vi "Main.vi"() -> ()   [LabVIEW 2020]
doc: "Cet exemple de projet Mesure continue est basé sur le modèle Gestionnaire de messages dans une file d'attente.\n\nLa boucle de gestion d'événements génère des messages en fonction des actions sur l'interface utilisateur.\n\nLa boucle de gestion de messages traite les messages générés par la boucle de gestion d'événements ou par d'autres messages. Il y a aussi des sous-VIs de boucle de gestion de messages d'acquisition et d'enregistrement, ainsi qu'une boucle de mise à jour du graphe déroulant."
uses:
  Settings/Settings.ctl
  Acquisition/Hardware Configuration.ctl
  Acquisition/Signal Type.ctl
  Logging/Logging Configuration.ctl
  controls/UI Data.ctl
  controls/UI State.ctl
  support/Message Queue/Enqueue Message (Single).vi
  support/Message Queue/Enqueue Message (Array).vi
  <vilib>/Utility/error.llb/Error Cluster From Error Code.vi
  <vilib>/ErrorRing/Error Ring.xnode
  Acquisition/Acquisition.lvlib
  Logging/Logging.lvlib
  Settings/Settings.lvlib
  support/User Event - Stop/User Event - Stop.lvlib
  support/Message Queue/Message Queue.lvlib
  Settings/Settings Dialog.vi
panel:
  in  "Panneaux":T1(tab)
  in  "Param status":bool
  out "Données":waveform(dbl)[](graph)
  out "État":string
  in  "Quitter":bool
  in  "Arrêter":bool
  in  "Démarrer":bool
  in  "Paramètres":bool
  # "MAPA Tech"
  # "MAPA Tech"
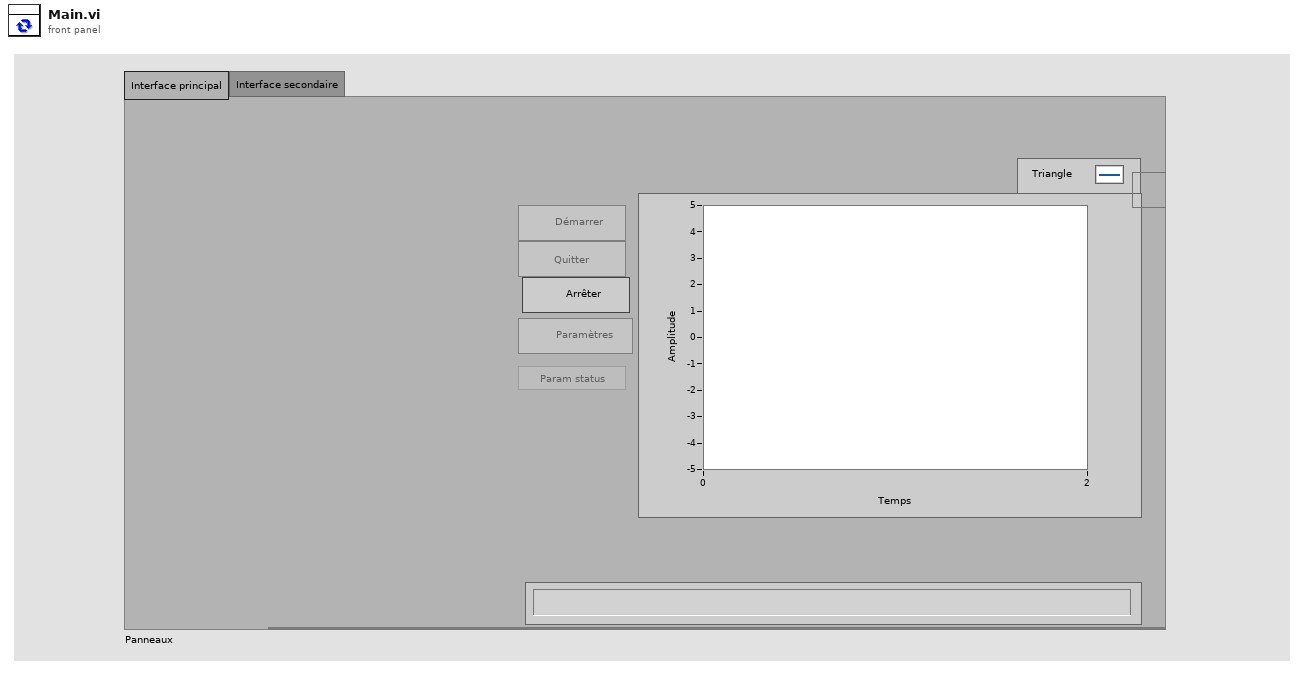
[diagram p1: front panel]
types:
  T1 = enum32{"Interface principal", "Interface secondaire"}
  T2 = typedef "UI State.ctl" = enum16{"Idle", "Acquiring and Logging", "Waiting for Exit", "Waiting for Exit (Acq Stopped)", "Waiting for Exit (Log Stopped)", "Waiting for Stop", "Waiting for Stop (Acq Stopped)", "Waiting for Stop (Log Stopped)"}
  T3 = typedef "UI Data.ctl" = cluster{"Réf. de Démarrer":refnum<vi>, "Réf. d'Arrêter":refnum<vi>, "Réf. de Paramètres":refnum<vi>, "Réf. de Quitter":refnum<vi>, "Réf. d'état":refnum<vi>, "Réf. de données":refnum<vi>, "Ref. Moyennage sélectionneur":refnum<vi>, "Ref. Param status":refnum<vi>}
  T4 = typedef "Settings.lvlib/Settings.ctl" = cluster{"Configuration du matériel":T5, "Configuration de l'enregistrement":T7, "Mode de longueur d'onde":cluster{"Choix du mode":bool, "Commande numérique":dbl}}
  T5 = typedef "Acquisition.lvlib/Hardware Configuration.ctl" = cluster{"Refnum de matériel <À remplacer>":string, "Type de signal <À remplacer>":T6}
  T6 = typedef "Acquisition.lvlib/Signal Type.ctl" = enum16{"Sine Wave", "Square with Noise", "Signal triangulaire", "Simulation DAQ"}
  T7 = typedef "Logging.lvlib/Logging Configuration.ctl" = cluster{"Chemin de base du fichier journal":path, "Référence de fichier TDMS":refnum<k34>}
  T8 = cluster{"état":bool, "code":i32, "source":string}
  T9 = typedef "Message Queue.lvlib/All Message Queues.ctl" = cluster{"IU":refnum<queue>, "Acquisition":refnum<queue>, "Enregistrement":refnum<queue>}
  T10 = cluster{"Choix du mode":bool, "Commande numérique":dbl}
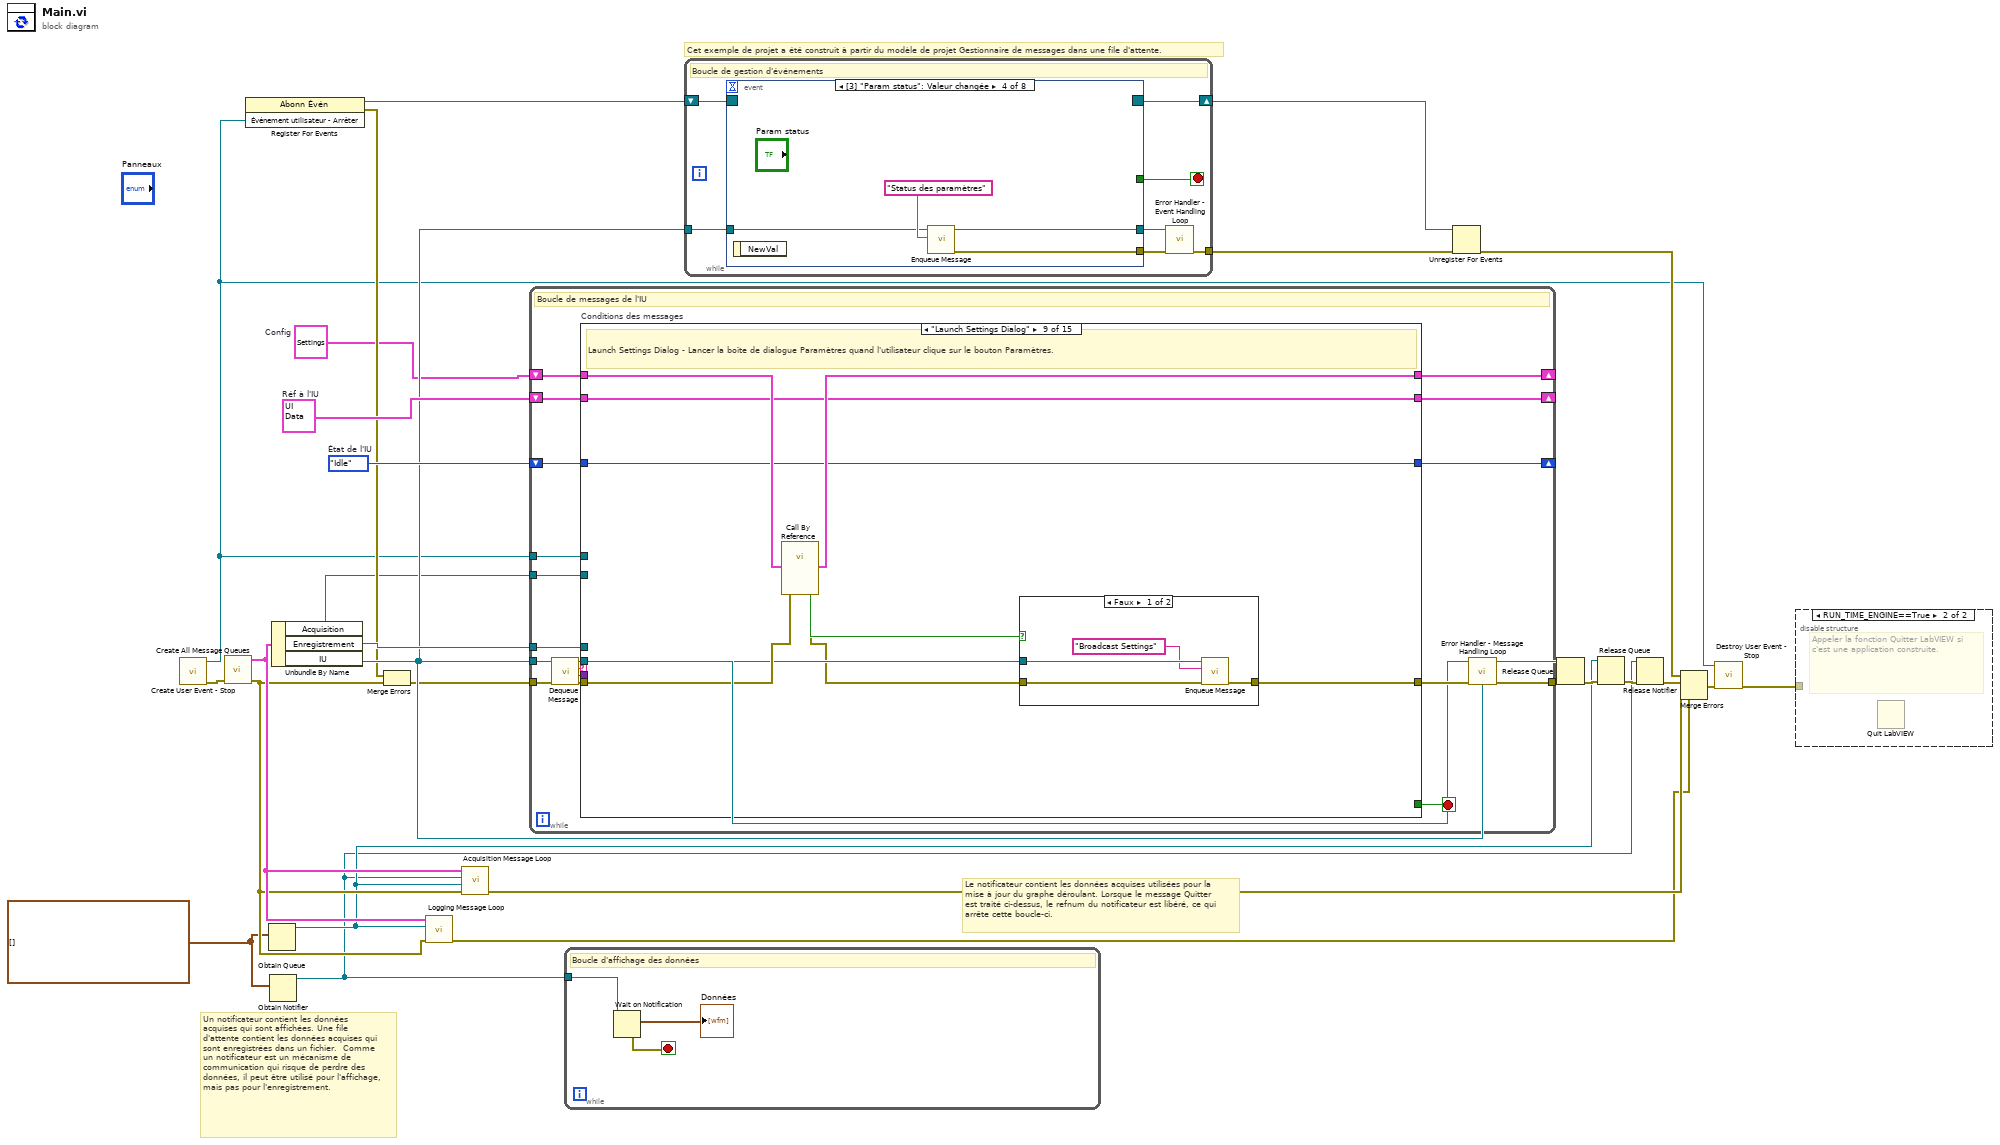
[diagram p0: block diagram]
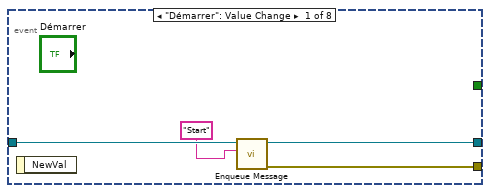
[diagram p3: hidden frame]
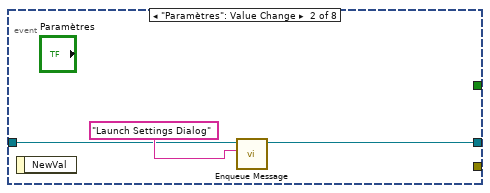
[diagram p4: hidden frame]
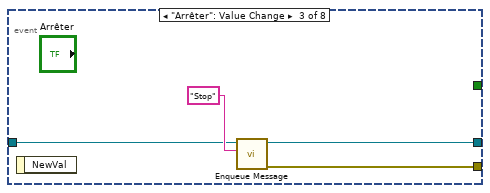
[diagram p5: hidden frame]
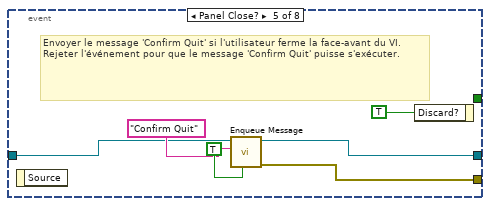
[diagram p6: hidden frame]
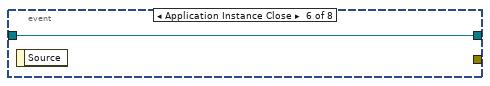
[diagram p7: hidden frame]
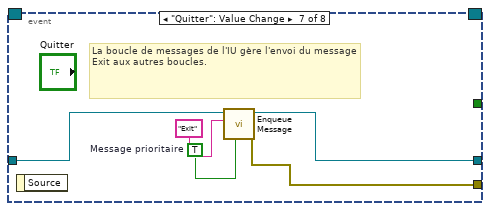
[diagram p8: hidden frame]
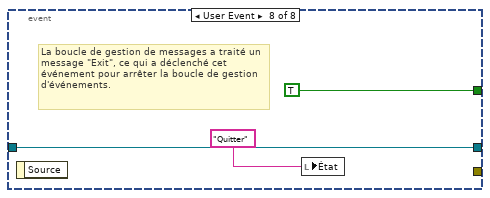
[diagram p9: hidden frame]
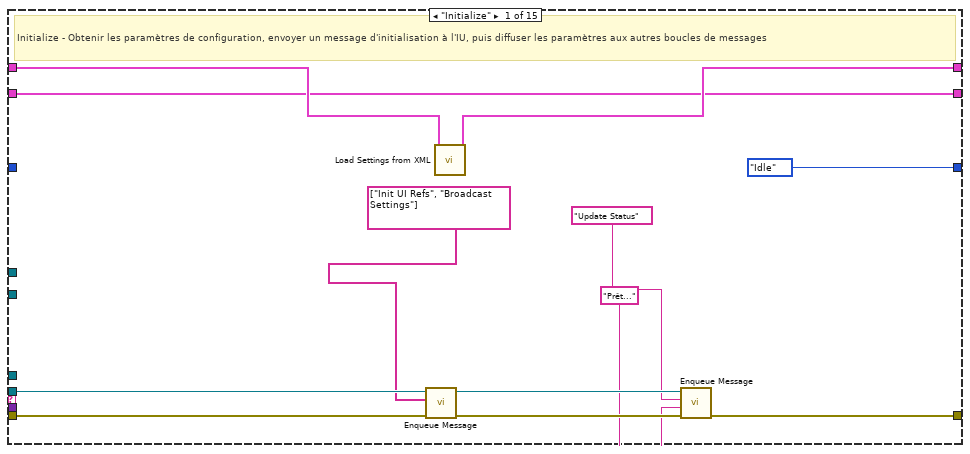
[diagram p10: hidden frame]
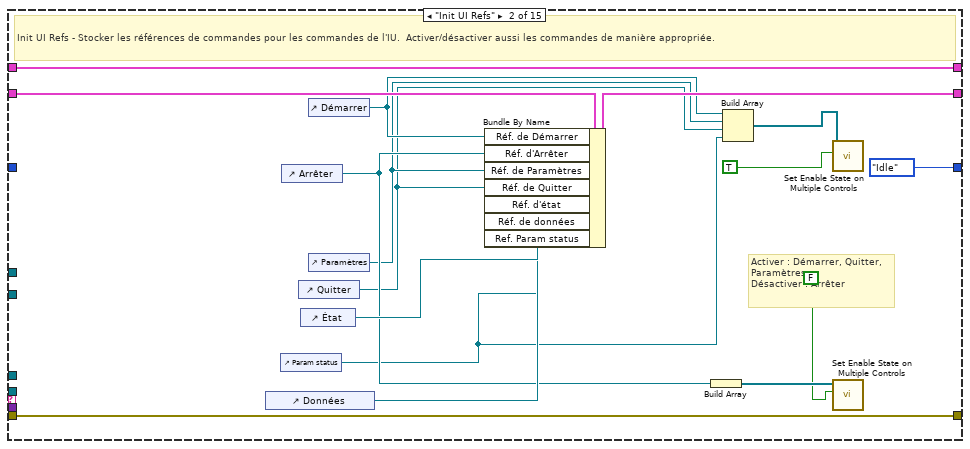
[diagram p11: hidden frame]
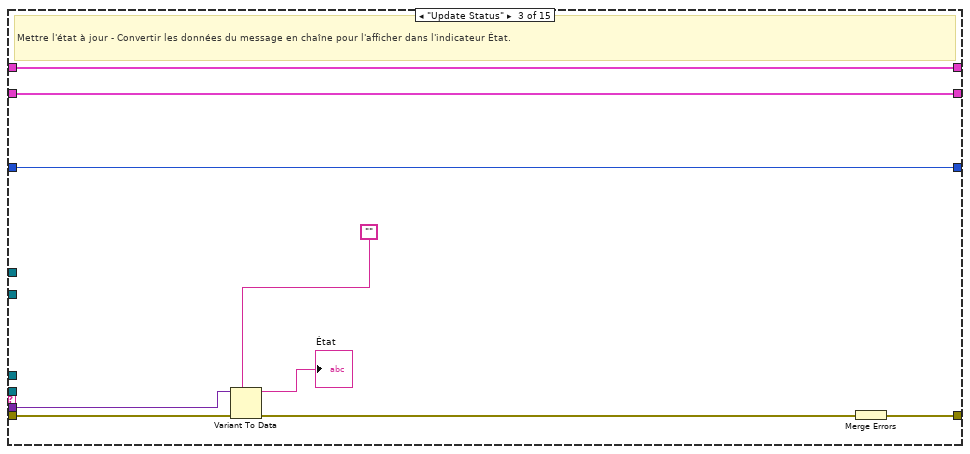
[diagram p12: hidden frame]
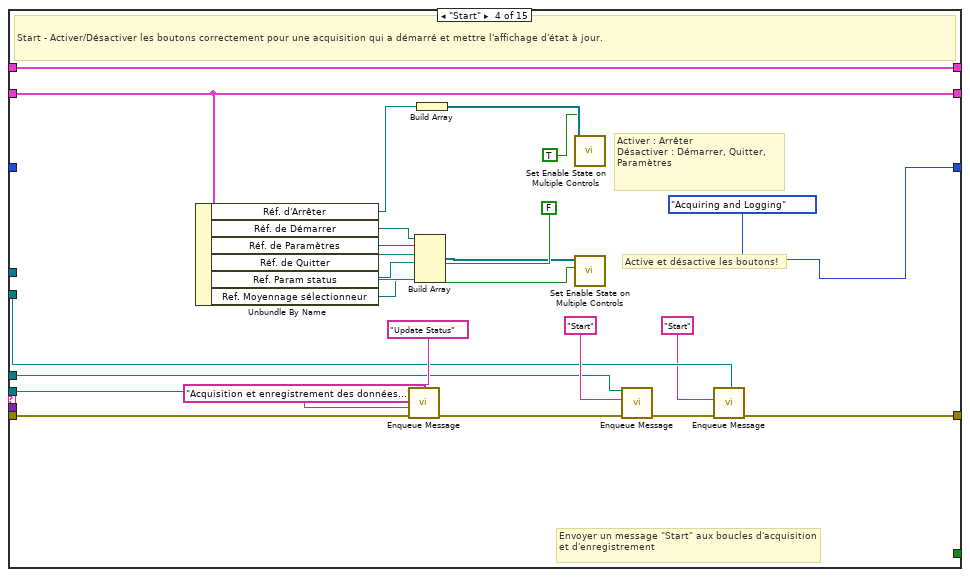
[diagram p13: hidden frame]
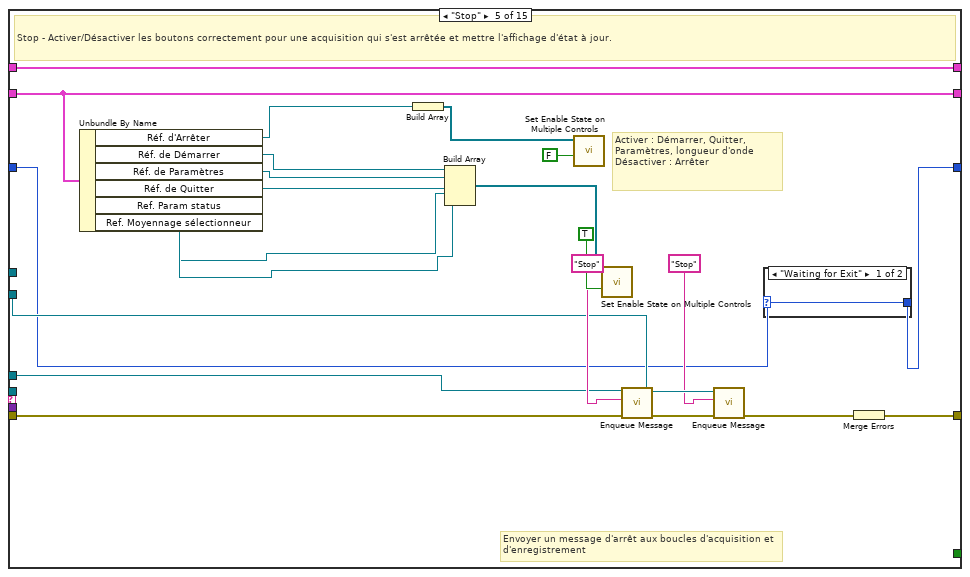
[diagram p14: hidden frame]
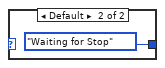
[diagram p15: hidden frame]
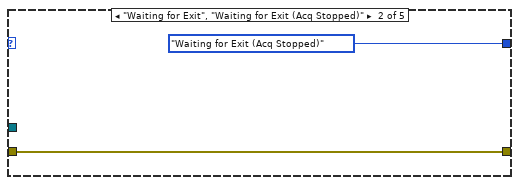
[diagram p17: hidden frame]
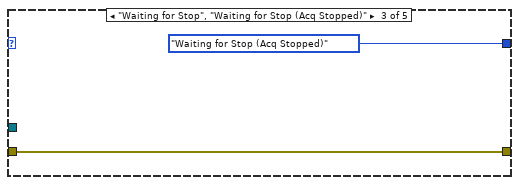
[diagram p18: hidden frame]
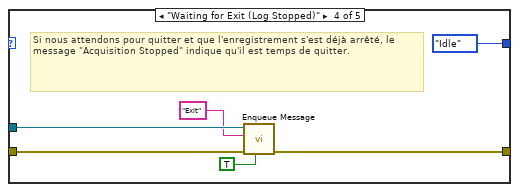
[diagram p19: hidden frame]
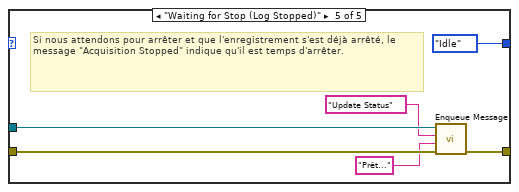
[diagram p20: hidden frame]
diagram:
  w16 = UI_State."Idle"  # État de l'IU
  w2 = waveform(dbl)[] []
  w18 = T3 {"Réf. de Démarrer"=refnum, "Réf. d'Arrêter"=refnum, "Réf. de Paramètres"=refnum, "Réf. de Quitter"=refnum, "Réf. d'état"=refnum, "Réf. de données"=refnum, "Ref. Moyennage sélectionneur"=refnum, "Ref. Param status"=refnum}  # Réf à l'IU
  w1 = T4 {"Configuration du matériel"={"Refnum de matériel <À remplacer>"="", "Type de signal <À remplacer>"=enum."Simulation DAQ"}, "Configuration de l'enregistrement"={"Chemin de base du fichier journal"=path "", "Référence de fichier TDMS"=refnum}, "Mode de longueur d'onde"={"Choix du mode"=TRUE, "Commande numérique"=15.0}}  # Config
  # "Cet exemple de projet a été construit à partir du modèle de projet Gestionnaire de messages dans une file d'attente."
  # "Un notificateur contient les données acquises qui sont affichées. Une file d'attente contient les données acquises qui sont enregistrées dans un fichier.  Comme un notificateur est un mécanisme de communication qui risque de perdre des données, il peut être utilisé pour l'affichage, mais pas pour l'enregistrement."
  # "Le notificateur contient les données acquises utilisées pour la mise à jour du graphe déroulant. Lorsque le message Quitter est traité ci-dessus, le refnum du notificateur est libéré, ce qui arrête cette boucle-ci."
  n1 = call "Create User Event - Stop.vi"() -> ("error out"=w24:T8, "Événement utilisateur - Arrêter"=w3:refnum<user-event>)  [unwired: 10 in]
  n2 = call "Create All Message Queues.vi"("error in (no error)"=w24) -> ("error out"=w21:T8, "Files d'attente de messages en sortie"=w23:T9)  [unwired: 9 in]
  n3 = register-events(w3) -> (reference out=w7:refnum<event-registration>, error out=w5:errorcluster)  [unwired: 2 in]
  n4 = Obtain Queue(element data type=w2) -> (queue out=w9:refnum<queue>)  [unwired: 4 in, 2 out]
  n5 = Obtain Notifier(notification data type=w2) -> (notifier out=w8:refnum<notifier>)  [unwired: 3 in, 2 out]
  n6 = Unbundle By Name(w23) -> ("Acquisition"=w4:refnum<queue>, "Enregistrement"=w17:refnum<queue>, "IU"=w14:refnum<queue>)
  n7 = Merge Errors(w5, w21) -> (w6:errorcluster)
  n8 = call "Logging Message Loop.vi"("error in (no error)"=w21, "File d'attente de données"=w9, "Files d'attente de messages"=w23) -> ("error out"=w22:T8)  [unwired: 8 in]
  n9 = call "Acquisition Message Loop.vi"("error in (no error)"=w21, "File d'attente de données"=w9, "Notificateur de données"=w8, "Files d'attente de messages"=w23) -> ("error out"=w25:T8)  [unwired: 7 in]
  n10 = while {
    tunnel: w14 -> [w39]
    tunnel: w3 -> [w44]
    shift-right: [w38] -> _
    shift-left: w1 -> [w37]
    shift-right: [w35] -> _
    shift-left: w18 -> [w36]
    tunnel: w4 -> [w34]
    tunnel: w17 -> [w33]
    shift-right: [w28] -> _
    shift-left: w16 -> [w29]
    tunnel: w6 -> [w43]
    tunnel: [w32] -> w27
    stop <- w45 stop-if-true
    # "Boucle de messages de l'IU"
    n11 = call "Dequeue Message.vi"("error in (no error)"=w43, "File d'attente de messages"=w39) -> ("error out"=w42:T8, "Données de message"=w40:variant, "Message"=w41:string, "File d'attente de message dup."=w30:refnum<queue>)  [unwired: 6 in]
    n12 = case "Conditions des messages" shown="\"Launch Settings Dialog\"" w41 {
      selector: w41 -> [_ _ _ _ _ _ _ _ _ _ _ _ _ _ w285]
      tunnel: w30 -> [w49 _ _ w106 _ w133 w158 _ w200 _ w221 _ _ w272 _]
      tunnel: w42 -> [w48 w73 w81 w105 w127 w134 w159 w188 w202 w209 w220 w249 w266 w276 _]
      tunnel: [w53 w73 w82 w92 w128 w131 w156 w194 w195 w212 w219 w259 w265 w275 w284] -> w31
      tunnel: [_ _ _ _ _ _ _ _ _ _ _ TRUE _ _ _] -> w45
      tunnel: w40 -> [_ _ w80 _ _ _ _ _ _ w213 _ w247 _ _ _]
      tunnel: w44 -> [_ _ _ _ _ _ _ _ _ _ _ w260 _ _ _]
      tunnel: [w56 w72 w76 w104 w126 w137 w162 w192 w199 w217 w224 w258 w264 w270 w288] -> w38
      tunnel: w37 -> [w57 w72 w76 w104 w126 w137 w162 w192 w203 w217 w224 w258 w264 w270 w288]
      tunnel: w36 -> [w50 w71 w75 w101 w125 w136 w161 w187 w197 w216 w223 w257 w263 w274 w287]
      tunnel: [w50 w68 w75 w101 w125 w136 w161 w187 w197 w216 w223 w257 w263 w274 w287] -> w35
      tunnel: w34 -> [_ _ _ w91 w118 _ _ w186 _ _ _ w256 _ _ _]
      tunnel: w33 -> [_ _ _ w94 w121 _ _ w181 _ _ _ w255 _ _ _]
      tunnel: w29 -> [_ _ w74 _ w115 w135 w160 w185 w196 w211 w222 _ w262 _ w286]
      tunnel: [UI_State."Idle" ("UI State") UI_State."Idle" ("UI State") w74 UI_State."Acquiring and Logging" ("UI State") w116 w132 w157 w185 w196 w211 w218 UI_State."Idle" ("UI State") w262 UI_State."Acquiring and Logging" ("UI State") w286] -> w28
      frame "Initialize" {
        # "Initialize - Obtenir les paramètres de configuration, envoyer un message d'initialisation à l'IU, puis diffuser les paramètres aux autres boucles de messages"
        n13 = call-poly "Enqueue Message.vi"("error in (no error)"=w48, "Tableau de messages"=string[] ["Init UI Refs", "Broadcast Settings"], "File d'attente de messages"=w49) -> ("error out"=w55:T8, "File d'attente de message dup."=w54:refnum<queue>)  [unwired: 7 in]
        n14 = call "Load Settings from XML.vi"("Paramètres en entrée"=w57) -> ("Paramètres en sortie"=w56:T4)  [unwired: 9 in, 1 out]
        n15 = call-poly "Enqueue Message.vi"("error in (no error)"=w55, "Données de message"="Prêt..." ("Ready..."), "Message"="Update Status", "File d'attente de messages"=w54) -> ("error out"=w53:T8)  [unwired: 6 in, 1 out]
      }
      frame "Init UI Refs" {
        # "Activer : Démarrer, Quitter, Paramètres\nDésactiver : Arrêter"
        # "Init UI Refs - Stocker les références de commandes pour les commandes de l'IU.  Activer/désactiver aussi les commandes de manière appropriée."
        n16 = control-ref of="Données"() -> (w69:refnum<vi>)
        n17 = control-ref of="Param status"() -> (w58:refnum<vi>)
        n18 = control-ref of="Arrêter"() -> (w63:refnum<vi>)
        n19 = control-ref of="Quitter"() -> (w60:refnum<vi>)
        n20 = control-ref of="État"() -> (w70:refnum<vi>)
        n21 = control-ref of="Démarrer"() -> (w62:refnum<vi>)
        n22 = control-ref of="Paramètres"() -> (w61:refnum<vi>)
        n23 = Bundle By Name(cluster=w71, "Réf. de Démarrer"=w62, "Réf. d'Arrêter"=w63, "Réf. de Paramètres"=w61, "Réf. de Quitter"=w60, "Réf. d'état"=w70, "Réf. de données"=w69, "Ref. Param status"=w58) -> (w68:T3)
        n24 = Build Array(w63) -> (w65:refnum<vi>[])
        n25 = Build Array(w62, w61, w60, w58) -> (w66:refnum<vi>[])
        n26 = call "Set Enable State on Multiple Controls.vi"("Activé ?"=TRUE ("Enable?"), "Commandes"=w66) -> ()  [unwired: 10 in]
        n27 = call "Set Enable State on Multiple Controls.vi"("Activé ?"=FALSE ("Enable?"), "Commandes"=w65) -> ()  [unwired: 10 in]
      }
      frame "Update Status" {
        # "Mettre l'état à jour - Convertir les données du message en chaîne pour l'afficher dans l'indicateur État."
        n28 = Variant To Data(error in=w81, type="" ("Empty String Constant"), Variant=w80) -> (data=→"État":string, error out=w78:errorcluster)
        n29 = Merge Errors(w78) -> (w82:errorcluster)
      }
      frame "Start" {
        # "Active et désactive les boutons!"
        # "Envoyer un message \"Start\" aux boucles d'acquisition et d'enregistrement"
        # "Activer : Arrêter\nDésactiver : Démarrer, Quitter, Paramètres"
        # "Start - Activer/Désactiver les boutons correctement pour une acquisition qui a démarré et mettre l'affichage d'état à jour."
        n30 = Unbundle By Name(w101) -> ("Réf. d'Arrêter"=w83:refnum<vi>, "Réf. de Démarrer"=w84:refnum<vi>, "Réf. de Paramètres"=w85:refnum<vi>, "Réf. de Quitter"=w88:refnum<vi>, "Ref. Param status"=w87:refnum<vi>, "Ref. Moyennage sélectionneur"=w86:refnum<vi>)
        n31 = call-poly "Enqueue Message.vi"("error in (no error)"=w105, "Données de message"="Acquisition et enregistrement des données..." ("Acquiring and Logging..."), "Message"="Update Status", "File d'attente de messages"=w106) -> ("error out"=w96:T8)  [unwired: 6 in, 1 out]
        n32 = Build Array(w84, w85, w85, w88, w87, w86) -> (w99:refnum<vi>[])
        n33 = Build Array(w83) -> (w98:refnum<vi>[])
        n34 = call "Set Enable State on Multiple Controls.vi"("Activé ?"=TRUE ("Enable?"), "Commandes"=w98) -> ()  [unwired: 10 in]
        n35 = call "Set Enable State on Multiple Controls.vi"("Activé ?"=FALSE ("Enable?"), "Commandes"=w99) -> ()  [unwired: 10 in]
        n36 = call-poly "Enqueue Message.vi"("error in (no error)"=w96, "Message"="Start", "File d'attente de messages"=w94) -> ("error out"=w93:T8)  [unwired: 7 in, 1 out]
        n37 = call-poly "Enqueue Message.vi"("error in (no error)"=w93, "Message"="Start", "File d'attente de messages"=w91) -> ("error out"=w92:T8)  [unwired: 7 in, 1 out]
      }
      frame "Stop" {
        # "Envoyer un message d'arrêt aux boucles d'acquisition et d'enregistrement"
        # "Activer : Démarrer, Quitter, Paramètres, longueur d'onde\nDésactiver : Arrêter"
        # "Stop - Activer/Désactiver les boutons correctement pour une acquisition qui s'est arrêtée et mettre l'affichage d'état à jour."
        n38 = Unbundle By Name(w125) -> ("Réf. d'Arrêter"=w107:refnum<vi>, "Réf. de Démarrer"=w108:refnum<vi>, "Réf. de Paramètres"=w109:refnum<vi>, "Réf. de Quitter"=w110:refnum<vi>, "Ref. Param status"=w111:refnum<vi>, "Ref. Moyennage sélectionneur"=w112:refnum<vi>)
        n39 = Build Array(w107) -> (w113:refnum<vi>[])
        n40 = Build Array(w108, w109, w110, w111, w112) -> (w114:refnum<vi>[])
        n41 = call "Set Enable State on Multiple Controls.vi"("Activé ?"=FALSE ("Enable?"), "Commandes"=w113) -> ()  [unwired: 10 in]
        n42 = call "Set Enable State on Multiple Controls.vi"("Activé ?"=TRUE ("Enable?"), "Commandes"=w114) -> ()  [unwired: 10 in]
        n43 = call-poly "Enqueue Message.vi"("error in (no error)"=w127, "Message"="Stop", "File d'attente de messages"=w121) -> ("error out"=w120:T8)  [unwired: 7 in, 1 out]
        n44 = call-poly "Enqueue Message.vi"("error in (no error)"=w120, "Message"="Stop", "File d'attente de messages"=w118) -> ("error out"=w119:T8)  [unwired: 7 in, 1 out]
        n45 = case shown="\"Waiting for Exit\"" w115 {
          selector: w115 -> [w129 _]
          tunnel: [w129 UI_State."Waiting for Stop" ("UI State")] -> w116
          frame "Waiting for Exit" {
          }
          frame Default {
          }
        }
        n46 = Merge Errors(w119) -> (w128:errorcluster)
      }
      frame "Acquisition Stopped" {
        # "Logique déterminant quelle action entreprendre quand l'acquisition s'est arrêtée."
        n47 = case shown="Par défaut" w135 {
          selector: w135 -> [w139 _ _ _ _]
          tunnel: w134 -> [w138 w141 w143 w149 w155]
          tunnel: w133 -> [_ _ _ w147 w152]
          tunnel: [w139 UI_State."Waiting for Exit (Acq Stopped)" ("UI State") UI_State."Waiting for Stop (Acq Stopped)" ("UI State") UI_State."Idle" ("UI State") UI_State."Idle" ("UI State")] -> w132
          tunnel: [w138 w141 w143 w148 w153] -> w131
          frame Default {
          }
          frame "Waiting for Exit", "Waiting for Exit (Acq Stopped)" {
          }
          frame "Waiting for Stop", "Waiting for Stop (Acq Stopped)" {
          }
          frame "Waiting for Exit (Log Stopped)" {
            # "Si nous attendons pour quitter et que l'enregistrement s'est déjà arrêté, le message \"Acquisition Stopped\" indique qu'il est temps de quitter."
            n48 = call-poly "Enqueue Message.vi"("Message prioritaire ? (F)"=TRUE ("Priority Message? (F)"), "error in (no error)"=w149, "Message"="Exit", "File d'attente de messages"=w147) -> ("error out"=w148:T8)  [unwired: 6 in, 1 out]
          }
          frame "Waiting for Stop (Log Stopped)" {
            # "Si nous attendons pour arrêter et que l'enregistrement s'est déjà arrêté, le message \"Acquisition Stopped\" indique qu'il est temps d'arrêter."
            n49 = call-poly "Enqueue Message.vi"("error in (no error)"=w155, "Données de message"="Prêt..." ("Ready..."), "Message"="Update Status", "File d'attente de messages"=w152) -> ("error out"=w153:T8)  [unwired: 6 in, 1 out]
          }
        }
      }
      frame "Logging Stopped" {
        # "Logique déterminant quelle action entreprendre quand l'enregistrement s'est arrêté."
        n50 = case shown="\"Waiting for Stop (Acq Stopped)\"" w160 {
          selector: w160 -> [w164 _ _ _ _]
          tunnel: w159 -> [w163 w166 w168 w174 w177]
          tunnel: w158 -> [_ _ _ w172 w176]
          tunnel: [w164 UI_State."Waiting for Exit (Log Stopped)" ("UI State") UI_State."Waiting for Stop (Log Stopped)" ("UI State") UI_State."Idle" ("UI State") UI_State."Idle" ("UI State")] -> w157
          tunnel: [w163 w166 w168 w173 w175] -> w156
          frame Default {
          }
          frame "Waiting for Exit", "Waiting for Exit (Log Stopped)" {
          }
          frame "Waiting for Stop", "Waiting for Stop (Log Stopped)" {
          }
          frame "Waiting for Exit (Acq Stopped)" {
            # "Si nous attendons pour quitter et que l'acquisition s'est déjà arrêtée, le message \"Logging Stopped\" indique qu'il est temps de quitter."
            n51 = call-poly "Enqueue Message.vi"("Message prioritaire ? (F)"=TRUE ("Priority Message? (F)"), "error in (no error)"=w174, "Message"="Exit", "File d'attente de messages"=w172) -> ("error out"=w173:T8)  [unwired: 6 in, 1 out]
          }
          frame "Waiting for Stop (Acq Stopped)" {
            # "Si nous attendons pour arrêter et que l'acquisition s'est déjà arrêtée, le message \"Logging Stopped\" indique qu'il est temps d'arrêter."
            n52 = call-poly "Enqueue Message.vi"("error in (no error)"=w177, "Données de message"="Prêt..." ("Ready..."), "Message"="Update Status", "File d'attente de messages"=w176) -> ("error out"=w175:T8)  [unwired: 6 in, 1 out]
          }
        }
      }
      frame "Broadcast settings" {
        w182 = "Update Settings" ("Message")
        # "Broadcast settings - Envoyer le message 'Update Settings' aux boucles de messages d'enregistrement et d'acquisition."
        n53 = Unbundle By Name(w192) -> ("Configuration du matériel"=w191:T5, "Configuration de l'enregistrement"=w190:T7, "Mode de longueur d'onde"=w184:T10)
        n54 = call-poly "Enqueue Message.vi"("Données de message"=w191, "Message"=w182, "File d'attente de messages"=w186) -> ("error out"=w193:T8)  [unwired: 7 in, 1 out]
        n55 = call-poly "Enqueue Message.vi"("Données de message"=w184, "Message"=w182, "File d'attente de messages"=w181) -> ("error out"=w183:T8)  [unwired: 7 in, 1 out]
        n56 = call-poly "Enqueue Message.vi"("error in (no error)"=w193, "Données de message"=w190, "Message"=w182, "File d'attente de messages"=w181) -> ("error out"=w189:T8)  [unwired: 6 in, 1 out]
        n57 = Merge Errors(w183, w189, w188) -> (w194:errorcluster)
      }
      frame "Launch Settings Dialog" {
        # "Launch Settings Dialog - Lancer la boîte de dialogue Paramètres quand l'utilisateur clique sur le bouton Paramètres."
        n58 = call-by-ref "?"("error in (no error)"=w202, "Paramètres en entrée"=w203) -> ("error out"=w198:T8, "Annulation ?"=w201:bool, "Paramètres en sortie"=w199:T4)  [unwired: 8 in, 3 out]
        n59 = case shown="Faux" w201 {
          tunnel: w200 -> [w207 _]
          tunnel: w198 -> [w206 w208]
          tunnel: [w205 w208] -> w195
          frame False {
            n60 = call-poly "Enqueue Message.vi"("error in (no error)"=w206, "Message"="Broadcast Settings", "File d'attente de messages"=w207) -> ("error out"=w205:T8)  [unwired: 7 in, 1 out]
          }
          frame True {
          }
        }
      }
      frame "Error" {
        # "Error - Afficher une boîte de dialogue d'erreur. Ce message est envoyé par les VIs \"Error Handler\" à la fin de l'exécution de chaque boucle de cette application."
        n61 = Variant To Data(error in=w209, type=errorcluster {"status"=FALSE, "code"=0, "source"=""} ("error constant"), Variant=w213) -> (data=w210:errorcluster, error out=w214:errorcluster)
        n62 = call <vilib>:"Simple Error Handler.vi"("error in (no error)"=w210) -> ()  [unwired: 4 in, 5 out]
        n63 = Merge Errors(w214) -> (w212:errorcluster)
      }
      frame "Confirm Quit" {
        # "Confirm Quit - Message qui confirme si l'utilisateur voulait vraiment quitter l'application."
        n64 = case shown="\"Acquiring and Logging\"" w222 {
          tunnel: w221 -> [w230 w234]
          tunnel: w220 -> [w229 w233]
          tunnel: [w228 w232] -> w219
          tunnel: [UI_State."Idle" ("UI State") w231] -> w218
          frame Default {
            # "Si 'Confirm Quit' survient alors que le système est inactif, le message de confirmation est inutile."
            n65 = call-poly "Enqueue Message.vi"("Message prioritaire ? (F)"=TRUE ("Priority Message? (F)"), "error in (no error)"=w229, "Message"="Exit", "File d'attente de messages"=w230) -> ("error out"=w228:T8)  [unwired: 6 in, 1 out]
          }
          frame "Acquiring and Logging" {
            n66 = Two Button Dialog(message="Voulez-vous vraiment quitter en cours d'acquisition ?" ("Confirm Quit Message"), 1:"Non" ("No"), 2:"Oui" ("Yes")) -> (T button?=w235:bool)
            n67 = case shown="Vrai" w235 {
              tunnel: w234 -> [_ w244]
              tunnel: w233 -> [w240 w245]
              tunnel: [w240 w243] -> w232
              tunnel: [UI_State."Acquiring and Logging" ("UI State") UI_State."Waiting for Exit" ("UI State")] -> w231
              frame False {
                # "L'utilisateur ne voulait pas quitter."
              }
              frame True {
                n68 = call-poly "Enqueue Message.vi"("error in (no error)"=w245, "Message"="Stop", "File d'attente de messages"=w244) -> ("error out"=w243:T8)  [unwired: 7 in, 1 out]
              }
            }
          }
        }
      }
      frame "Exit" {
        w251 = TRUE ("Priority Message? (F)")
        w252 = "Exit" ("Message")
        # "Afficher une boîte de dialogue d'erreur si 'Exit' a été appelé suite à une erreur."
        # "Arrêter le VI"
        # "Exit - Envoyer des messages Exit aux boucles d'acquisition et d'enregistrerment, et déclencher l'événement utilisateur pour arrêter la boucle de gestion d'événements."
        n69 = Variant To Data(type=errorcluster {"status"=FALSE, "code"=0, "source"=""} ("error constant"), Variant=w247) -> (data=w246:errorcluster)  [unwired: 1 in, 1 out]
        n70 = call <vilib>:"Simple Error Handler.vi"("error in (no error)"=w246) -> ()  [unwired: 4 in, 5 out]
        n71 = call-poly "Enqueue Message.vi"("Message prioritaire ? (F)"=w251, "error in (no error)"=w249, "Message"=w252, "File d'attente de messages"=w256) -> ("error out"=w253:T8)  [unwired: 6 in, 1 out]
        n72 = call-poly "Enqueue Message.vi"("Message prioritaire ? (F)"=w251, "error in (no error)"=w253, "Message"=w252, "File d'attente de messages"=w255) -> ("error out"=w250:T8)  [unwired: 6 in, 1 out]
        n73 = call "Fire User Event - Stop.vi"("error in (no error)"=w250, "Événement utilisateur - Arrêt"=w260) -> ("error out"=w259:T8)  [unwired: 9 in]
      }
      frame "---Copy This Frame---" {
        # "Dupliquez cette étape pour créer de nouveaux messages.  Changez ce commentaire dans l'étape dupliquée pour décrire ce message."
        n74 = Merge Errors(w266) -> (w265:errorcluster)
      }
      frame "Status des paramètres" {
        # "Dupliquez cette étape pour créer de nouveaux messages.  Changez ce commentaire dans l'étape dupliquée pour décrire ce message."
        n75 = Unbundle By Name(w270) -> ("Mode de longueur d'onde.Choix du mode"=w269:bool, "Mode de longueur d'onde.Commande numérique"=w268:dbl)
        n76 = case shown="Vrai" w269 {
          tunnel: [w277 w282] -> w267
          tunnel: w268 -> [_ w283]
          frame False {
            n77 = Concatenate Strings ("Concaténer des chaînes")("Status: Mode automatique") -> (w277:string)
          }
          frame True {
            n78 = Number To Decimal String(number=w283) -> (decimal integer string=w280:string)  [unwired: 1 in]
            n79 = Concatenate Strings ("Concaténer des chaînes")("Status: Mode manuel et la longueur d'onde sélectionnée est ", w280, " nm.") -> (w282:string)
          }
        }
        n80 = Merge Errors(w276) -> (w275:errorcluster)
        n81 = call-poly "Enqueue Message.vi"("Données de message"=w267, "Message"="Update Status", "File d'attente de messages"=w272) -> ()  [unwired: 7 in, 2 out]
      }
      frame Default {
        # "La condition 'Par défaut' ne s'exécute que s'il y a un message qui n'est défini dans aucune des autres conditions.  Renvoyer une erreur de programmation."
        n82 = xnode ("Error Ring")("paramètre 0"=w285) -> ("sortie d'erreur"=w284:errorcluster)
      }
    }
    n83 = call "Error Handler - Message Handling Loop.vi"("error in (no error)"=w31, "File d'attente de messages"=w30) -> ("erreur en entrée dup."=w32:T8)  [unwired: 8 in, 1 out]
  }
  n84 = while "Data Display Loop" {
    tunnel: w8 -> [w297]
    stop <- w298 stop-if-true
    # "Boucle d'affichage des données"
    n85 = Wait on Notification(notifier=w297) -> (notification=→"Données":waveform(dbl)[], error out=w298:errorcluster)  [unwired: 3 in, 2 out]
  }
  n86 = while {
    tunnel: w14 -> [w304]
    tunnel: [w301] -> w26
    shift-right: [w303] -> w19
    shift-left: w7 -> [w305]
    stop <- w302 stop-if-true
    # "Boucle de gestion d'événements"
    n87 = event shown="[3] \"Param status\": Valeur changée" {
      selector: w305 -> [_ _ _ _ _ _ _ _]
      dyn-events: [_ _ _ _ _ _ _ _] -> w303
      timeout: _ -> [_ _ _ _ _ _ _ _]
      tunnel: [_ _ _ _ _ _ _ TRUE ("Discard?")] -> w302
      tunnel: w304 -> [w309 w311 w315 w319 w324 w327 w329 w333]
      tunnel: [w307 _ w314 w318 w322 _ w332 _] -> w300
      tunnel: [w306 w310 w313 w317 w323 w327 w328 w333] -> w299
      event "Démarrer": Value Change {
        n88 = event-data() -> ()  [unwired: 1 in, 1 out]
        n89 = call-poly "Enqueue Message.vi"("Message"="Start", "File d'attente de messages"=w309) -> ("error out"=w307:T8, "File d'attente de message dup."=w306:refnum<queue>)  [unwired: 8 in]
      }
      event "Paramètres": Value Change {
        n90 = event-data() -> ()  [unwired: 1 in, 1 out]
        n91 = call-poly "Enqueue Message.vi"("Message"="Launch Settings Dialog", "File d'attente de messages"=w311) -> ("File d'attente de message dup."=w310:refnum<queue>)  [unwired: 8 in, 1 out]
      }
      event "Arrêter": Value Change {
        n92 = event-data() -> ()  [unwired: 1 in, 1 out]
        n93 = call-poly "Enqueue Message.vi"("Message"="Stop", "File d'attente de messages"=w315) -> ("error out"=w314:T8, "File d'attente de message dup."=w313:refnum<queue>)  [unwired: 8 in]
      }
      event "Param status": Value Change {
        n94 = event-data() -> ()  [unwired: 1 in, 1 out]
        n95 = call-poly "Enqueue Message.vi"("Message"="Status des paramètres", "File d'attente de messages"=w319) -> ("error out"=w318:T8, "File d'attente de message dup."=w317:refnum<queue>)  [unwired: 8 in]
      }
      event Panel Close? {
        # "Envoyer le message 'Confirm Quit' si l'utilisateur ferme la face-avant du VI. Rejeter l'événement pour que le message 'Confirm Quit' puisse s'exécuter."
        n96 = event-data() -> ()  [unwired: 1 in, 1 out]
        n97 = call-poly "Enqueue Message.vi"("Message prioritaire ? (F)"=TRUE ("Priority Message? (F)"), "Message"="Confirm Quit", "File d'attente de messages"=w324) -> ("error out"=w322:T8, "File d'attente de message dup."=w323:refnum<queue>)  [unwired: 7 in]
        n98 = event-data ("Event Filter Node")("Discard?"=TRUE) -> ()  [unwired: 1 in, 1 out]
      }
      event Application Instance Close {
        n99 = event-data() -> ()  [unwired: 1 in, 1 out]
      }
      event "Quitter": Value Change {
        w330 = TRUE  # Message prioritaire
        # "La boucle de messages de l'IU gère l'envoi du message Exit aux autres boucles."
        n100 = event-data() -> ()  [unwired: 1 in, 1 out]
        n101 = call-poly "Enqueue Message.vi"("Message prioritaire ? (F)"=w330, "Message"="Exit", "File d'attente de messages"=w329) -> ("error out"=w332:T8, "File d'attente de message dup."=w328:refnum<queue>)  [unwired: 7 in]
      }
      event User Event {
        # "La boucle de gestion de messages a traité un message \"Exit\", ce qui a déclenché cet événement pour arrêter la boucle de gestion d'événements."
        n102 = event-data() -> ()  [unwired: 1 in, 1 out]
        n103 = local write "État"("Quitter" ("Exit String")) -> ()
      }
    }
    n104 = call "Error Handler - Event Handling Loop.vi"("error in (no error)"=w300, "File d'attente de messages"=w299) -> ("erreur en entrée dup."=w301:T8)  [unwired: 8 in, 1 out]
  }
  n105 = Unregister For Events(event registration refnum=w19, error in=w26) -> (error out=w20:errorcluster)
  n106 = Release Queue(queue=w14, error in (no error)=w27) -> (error out=w12:errorcluster)  [unwired: 1 in, 2 out]
  n107 = Release Queue(queue=w9, error in (no error)=w12) -> (error out=w11:errorcluster)  [unwired: 1 in, 2 out]
  n108 = Release Notifier(notifier=w8, error in (no error)=w11) -> (error out=w10:errorcluster)  [unwired: 1 in, 2 out]
  n109 = Merge Errors(w20, w10, w25, w22) -> (w15:errorcluster)
  n110 = call "Destroy User Event - Stop.vi"("error in (no error)"=w15, "Événement utilisateur - Arrêt"=w3) -> ("error out"=w13:T8)  [unwired: 9 in]
  n111 = disable-structure "Conditional Disable Structure" shown="RUN_TIME_ENGINE==True" {
    disable-tunnel: w13 -> [_ _]
    frame condition #0 (active) {
    }
    frame condition #1 {
      # "Appeler la fonction Quitter LabVIEW si c'est une application construite."
      n112 = Quit LabVIEW() -> ()  [unwired: 1 in]
    }
  }
